vi "Read State.vi"(8 "error in (no error)":errorcluster, 11 "ChirpV2 in":refnum<class "ChirpV2.lvclass">) -> (0 "error out":errorcluster, 2 "Enum":T1=enum."Initialization", 3 "ChirpV2 out":refnum<class "ChirpV2.lvclass">)   [LabVIEW 2014, in "ChirpV2.lvclass"]
uses:
  ChirpV2.lvclass
  StateV2.ctl
  ChirpV2.lvclass/ChirpV2.ctl
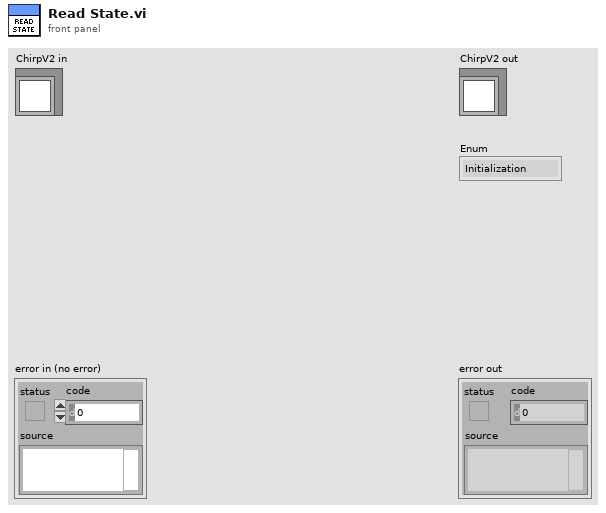
[diagram p1: front panel]
types:
  T1 = typedef "ChirpV2.lvclass/StateV2.ctl" = enum16{"WaitDC", "Initialization", "ChirpSetUp", "Wait", "ChirpMeasurement", "DFT", "WriteData", "Queue", "Ternimation"}
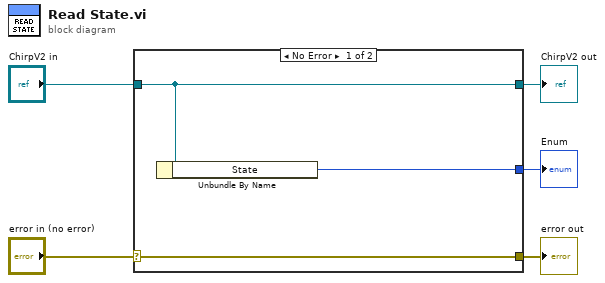
[diagram p0: block diagram]
diagram:
  n1 = case shown="No Error" "error in (no error)" {
    selector: "error in (no error)" -> [w8 w9]
    tunnel: [w8 w9] -> w4
    tunnel: [w7 w10] -> w2
    tunnel: "ChirpV2 in" -> [w7 w10]
    tunnel: [w6 _] -> w1
    frame No Error {
      n2 = Unbundle By Name(w7) -> ("State"=w6:T1)
    }
    frame Error {
    }
  }
  "error out" <- w4
  "ChirpV2 out" <- w2
  "Enum" <- w1
